vi "ReadPowerMulti.vi"(8 "error in":errorcluster, 9 "Config In":T1[](array[typedef]) {"Shunt Resistor" format="%#_g ohm"; "I2C"."Slave Address" format="%.0x"; "Calibration Value" format="%.0x"; "Mode" items=["Power Down", "Shunt Voltage, Triggered", "Bus Voltage, Triggered", "Shunt & Bus, Triggered", "ADC Off (Disabled)", "Shunt Voltage, Continuous", "Bus Voltage, Continuous", "Shunt & Bus Voltage, Continuous"]; "Shunt Voltage ADC Settings" items=["9-bit, 84us conversion time"=0, "10-bit, 148us conversion time"=1, "11-bit, 276us conversion time"=2, "12-bit, 532us conversion time"=3, "1x12-bit, 532us conversion time"=8, "2x12-bit averaged, 1.06ms conversion time"=9, "4x12-bit averaged, 2.13ms conversion time"=10, "8x12-bit averaged, 4.26ms conversion time"=11, "16x12-bit averaged, 8.51ms conversion time"=12, "32x12-bit averaged, 17.02ms conversion time"=13, "64x12-bit averaged, 34.05ms conversion time"=14, "128x12-bit averaged, 68.10ms conversion time"=15]; "Bus Voltage ADC Settings" items=["9-bit, 84us conversion time"=0, "10-bit, 148us conversion time"=1, "11-bit, 276us conversion time"=2, "12-bit, 532us conversion time"=3, "1x12-bit, 532us conversion time"=8, "2x12-bit averaged, 1.06ms conversion time"=9, "4x12-bit averaged, 2.13ms conversion time"=10, "8x12-bit averaged, 4.26ms conversion time"=11, "16x12-bit averaged, 8.51ms conversion time"=12, "32x12-bit averaged, 17.02ms conversion time"=13, "64x12-bit averaged, 34.05ms conversion time"=14, "128x12-bit averaged, 68.10ms conversion time"=15]; "PGA/Shunt Voltage Gain" items=["Gain 1, +/-40mV", "Gain 2, +/-80mV", "Gain 3, +/-160mV", "Gain 4, +/-320mV"]; "Bus Voltage Range" items=["0-16V Range", "0-32V Range"]; "Reset bit" items=["Do Not Reset", "Reset"]}) -> (0 "error out":errorcluster, 1 "Config Out":T1[](array[typedef]) {"Shunt Resistor" format="%#_g ohm"; "I2C"."Slave Address" format="%.0x"; "Calibration Value" format="%.0x"; "Mode" items=["Power Down", "Shunt Voltage, Triggered", "Bus Voltage, Triggered", "Shunt & Bus, Triggered", "ADC Off (Disabled)", "Shunt Voltage, Continuous", "Bus Voltage, Continuous", "Shunt & Bus Voltage, Continuous"]; "Shunt Voltage ADC Settings" items=["9-bit, 84us conversion time"=0, "10-bit, 148us conversion time"=1, "11-bit, 276us conversion time"=2, "12-bit, 532us conversion time"=3, "1x12-bit, 532us conversion time"=8, "2x12-bit averaged, 1.06ms conversion time"=9, "4x12-bit averaged, 2.13ms conversion time"=10, "8x12-bit averaged, 4.26ms conversion time"=11, "16x12-bit averaged, 8.51ms conversion time"=12, "32x12-bit averaged, 17.02ms conversion time"=13, "64x12-bit averaged, 34.05ms conversion time"=14, "128x12-bit averaged, 68.10ms conversion time"=15]; "Bus Voltage ADC Settings" items=["9-bit, 84us conversion time"=0, "10-bit, 148us conversion time"=1, "11-bit, 276us conversion time"=2, "12-bit, 532us conversion time"=3, "1x12-bit, 532us conversion time"=8, "2x12-bit averaged, 1.06ms conversion time"=9, "4x12-bit averaged, 2.13ms conversion time"=10, "8x12-bit averaged, 4.26ms conversion time"=11, "16x12-bit averaged, 8.51ms conversion time"=12, "32x12-bit averaged, 17.02ms conversion time"=13, "64x12-bit averaged, 34.05ms conversion time"=14, "128x12-bit averaged, 68.10ms conversion time"=15]; "PGA/Shunt Voltage Gain" items=["Gain 1, +/-40mV", "Gain 2, +/-80mV", "Gain 3, +/-160mV", "Gain 4, +/-320mV"]; "Bus Voltage Range" items=["0-16V Range", "0-32V Range"]; "Reset bit" items=["Do Not Reset", "Reset"]}, 2 "Power Readings":T2[](array[typedef]) {"Current" format="%#.3g A"; "Power" format="%#.3g W"; "Shunt Voltage" format=" %#.3g V"; "Bus Voltage" format="%#.3g V"; "Voltage (Total)" format="%#.3g V"})   [LabVIEW 2018]
uses:
  Sensors/Power Sensor - Adafruit INA219/INA219 Measurements.ctl
  Sensors/Power Sensor - Adafruit INA219/INA219 Config Options.ctl
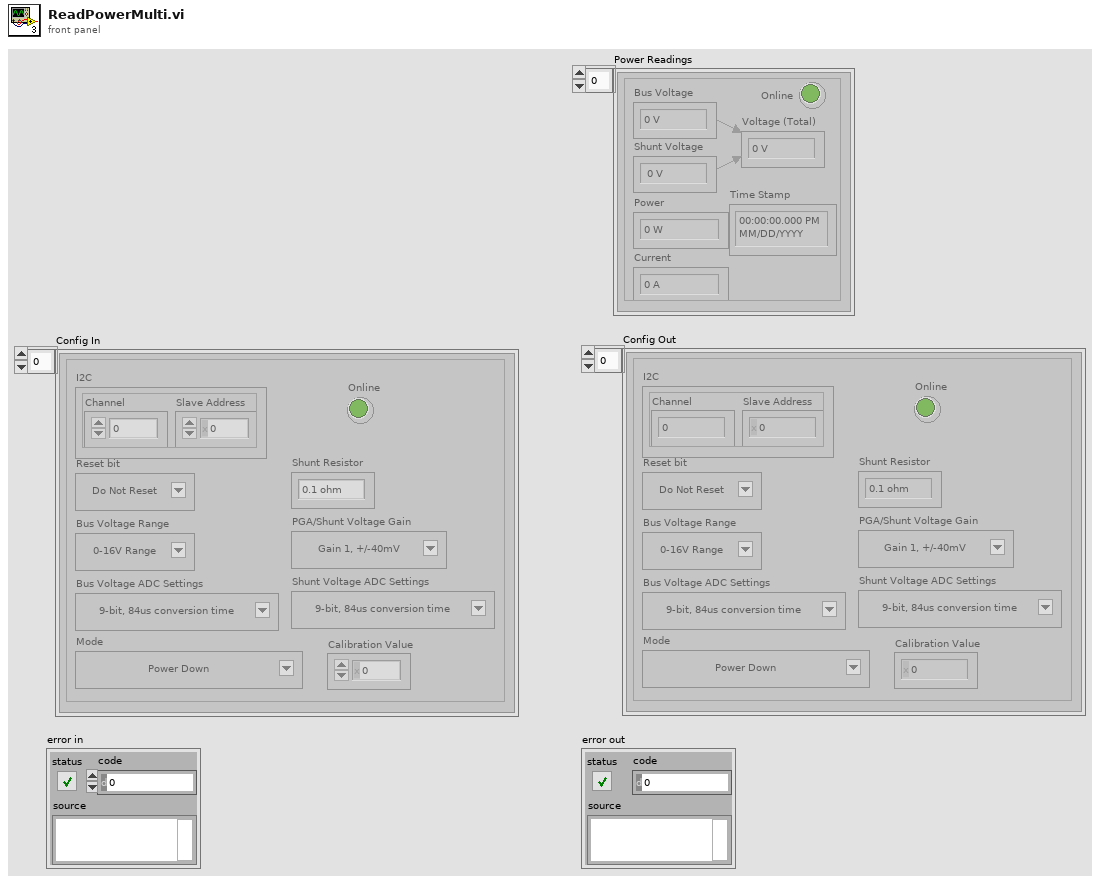
[diagram p1: front panel]
types:
  T1 = typedef "INA219 Config Options.ctl" = cluster{"I2C":cluster{"Slave Address":u8, "Channel":u8}, "Reset bit":u8, "Bus Voltage Range":u8, "PGA/Shunt Voltage Gain":u8, "Bus Voltage ADC Settings":u8, "Shunt Voltage ADC Settings":u8, "Mode":u8, "Calibration Value":u16, "Online":bool, "Shunt Resistor":dbl}
  T2 = typedef "INA219 Measurements.ctl" = cluster{"Voltage (Total)":dbl, "Bus Voltage":dbl, "Shunt Voltage":dbl, "Power":dbl, "Current":dbl, "Online":bool, "Time Stamp":timestamp}
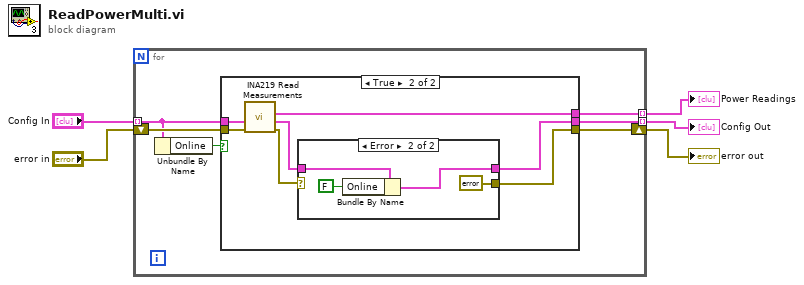
[diagram p0: block diagram]
diagram:
  n1 = for {
    tunnel: "Config In" -> [w7] mode=indexing
    shift-right: [w10] -> w3
    shift-left: "error in" -> [w11]
    tunnel: [w9] -> w4 mode=indexing
    tunnel: [w8] -> w5 mode=indexing
    n2 = Unbundle By Name(w7) -> ("Online"=w6:bool)
    n3 = case shown="True" w6 {
      tunnel: w11 -> [w12 w20]
      tunnel: w7 -> [w13 w18]
      tunnel: [w12 w14] -> w10
      tunnel: [w13 w16] -> w9
      tunnel: [_ w19] -> w8
      frame False {
      }
      frame True {
        n4 = call "INA219 Read Measurements.vi"("error in (no error)"=w20, "INA219 Config Options"=w18) -> ("error out"=w15:errorcluster, "INA219 Config Options"=w17:T1, "Measurements"=w19:T2)  [unwired: 6 in, 1 out]
        n5 = case shown="Error" w15 {
          selector: w15 -> [w21 _]
          tunnel: w17 -> [w22 w25]
          tunnel: [w22 w23] -> w16
          tunnel: [w21 errorcluster {"status"=FALSE, "code"=0, "source"=""} ("error IO")] -> w14
          frame No Error {
          }
          frame Error {
            n6 = Bundle By Name(cluster=w25, "Online"=FALSE) -> (w23:T1)
          }
        }
      }
    }
  }
  "Power Readings" <- w5
  "Config Out" <- w4
  "error out" <- w3
